vi "AlliGator_Graphs Metadata Types.vi"(11 "Graph Label":string) -> (1 "Found?":bool, 3 "Plot Metadata Type":variant)   [LabVIEW 2021, in "AlliGator GUI.lvlib"]
uses:
  AlliGator GUI.lvlib
  Lifetime & Other Parameters/AlliGator Lifetime & Other Parameters Plot Metadata.ctl
  Lifetime & Other Parameters/AlliGator Lifetime & Other Parameters.lvlib
panel:
  # "see the License on the block diagram (Ctrl+E or Window:Show Block Diagram)"
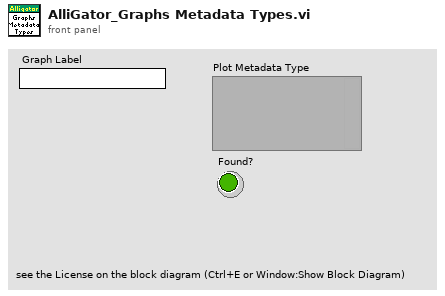
[diagram p1: front panel]
types:
  T1 = typedef "AlliGator Lifetime & Other Parameters.lvlib/AlliGator Lifetime & Other Parameters Plot Metadata.ctl" = cluster{"Intensity Array":dbl[]}
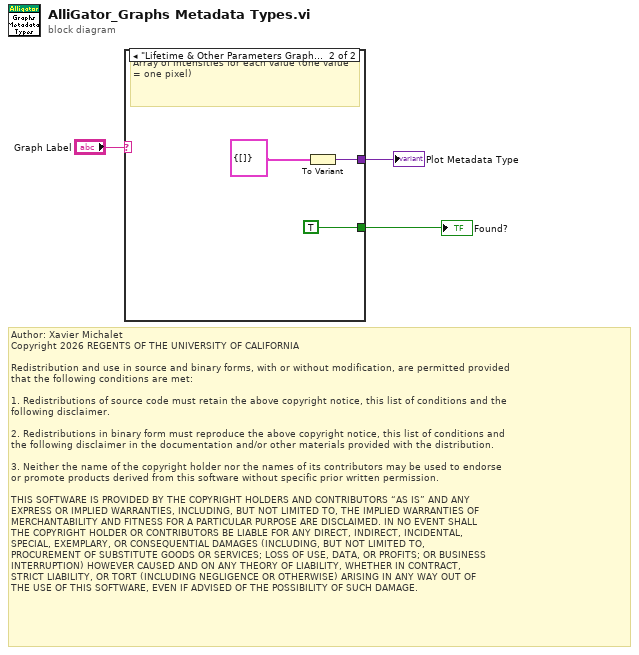
[diagram p0: block diagram]
diagram:
  # "Author: Xavier Michalet\nCopyright 2026 REGENTS OF THE UNIVERSITY OF CALIFORNIA\n\nRedistribution and use in source and binary forms, with or without modification, are permitted provided\nthat the following conditions are met:\n\n1. Redistributions of source code must retain the above copyright notice, this list of conditions and the\nfollowing disclaimer.\n\n2. Redistributions in binary form must reproduce the above copyright notice, this list of conditions and\nthe following disclaimer in the documentation and/or other materials provided with the distribution.\n\n3. Neither the name of the copyright holder nor the names of its contributors may be used to endorse \nor promote products derived from this software without specific prior written permission.\n\nTHIS SOFTWARE IS PROVIDED BY THE COPYRIGHT HOLDERS AND CONTRIBUTORS “AS IS” AND ANY \nEXPRESS OR IMPLIED WARRANTIES, INCLUDING, BUT NOT LIMITED TO, THE IMPLIED WARRANTIES OF\nMERCHANTABILITY AND FITNESS FOR A PARTICULAR PURPOSE ARE DISCLAIMED. IN NO EVENT SHALL\nTHE COPYRIGHT HOLDER OR CONTRIBUTORS BE LIABLE FOR ANY DIRECT, INDIRECT, INCIDENTAL, \nSPECIAL, EXEMPLARY, OR CONSEQUENTIAL DAMAGES (INCLUDING, BUT NOT LIMITED TO, \nPROCUREMENT OF SUBSTITUTE GOODS OR SERVICES; LOSS OF USE, DATA, OR PROFITS; OR BUSINESS\nINTERRUPTION) HOWEVER CAUSED AND ON ANY THEORY OF LIABILITY, WHETHER IN CONTRACT, \nSTRICT LIABILITY, OR TORT (INCLUDING NEGLIGENCE OR OTHERWISE) ARISING IN ANY WAY OUT OF\nTHE USE OF THIS SOFTWARE, EVEN IF ADVISED OF THE POSSIBILITY OF SUCH DAMAGE."
  n1 = case shown="\"Lifetime & Other Parameters Graph\"" "Graph Label" {
    tunnel: [_ w6] -> w2
    tunnel: [_ TRUE ("Found?")] -> w1
    frame "", Default {
    }
    frame "Lifetime & Other Parameters Graph" {
      # "Array of Intensities for each value (one value = one pixel)"
      n2 = To Variant(anything=T1 {"Intensity Array"=[]} ("Lifetime Plot Metadata")) -> (Variant=w6:variant)
    }
  }
  "Plot Metadata Type" <- w2
  "Found?" <- w1
